vi "Kommunikation Geraetekennung.vi"(8 "error in (no error)":errorcluster caption="Fehler (Eingang, kein Fehler)", 11 "Steuerung PNS Eingang":refnum<class "Steuerung PNS.lvclass">) -> (0 "error out":errorcluster caption="Fehler (Ausgang)", 1 "Seriennummer":string, 2 "Gerätetype":string, 3 "Steuerung PNS Ausgang":refnum<class "Steuerung PNS.lvclass">)   [LabVIEW 2020, in "Steuerung PNS.lvclass"]
doc: "Kommuniziert mit der Steuerung, um die GeräteType auszulesen und in die Typenbezeichnung umzuwandeln, speichert diese im Objekt und stellt sie gelichzeitig als Output zur Verfügung.\nRIW"
uses:
  Steuerung PNS.lvclass
panel:
  out "SoftWare Vresion":string
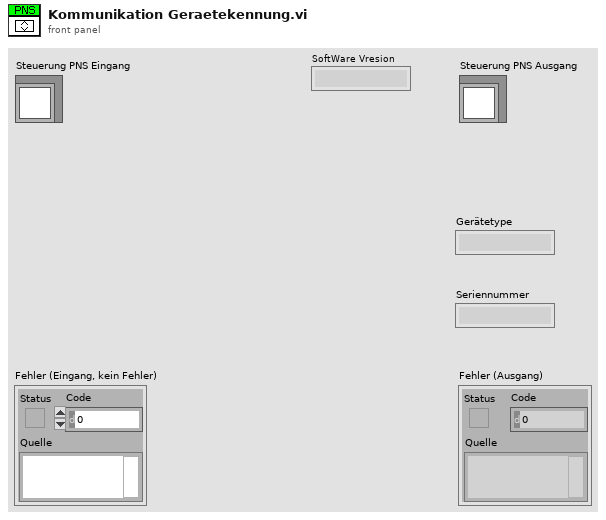
[diagram p1: front panel]
types:
  T1 = typedef "Steuerung PNS.lvclass/Adresse.ctl" = cluster{i32[][], i32}
  T2 = typedef "Steuerung PNS.lvclass/Werte.ctl" = cluster{"Adressen":u16[], "Werte":u16[]}
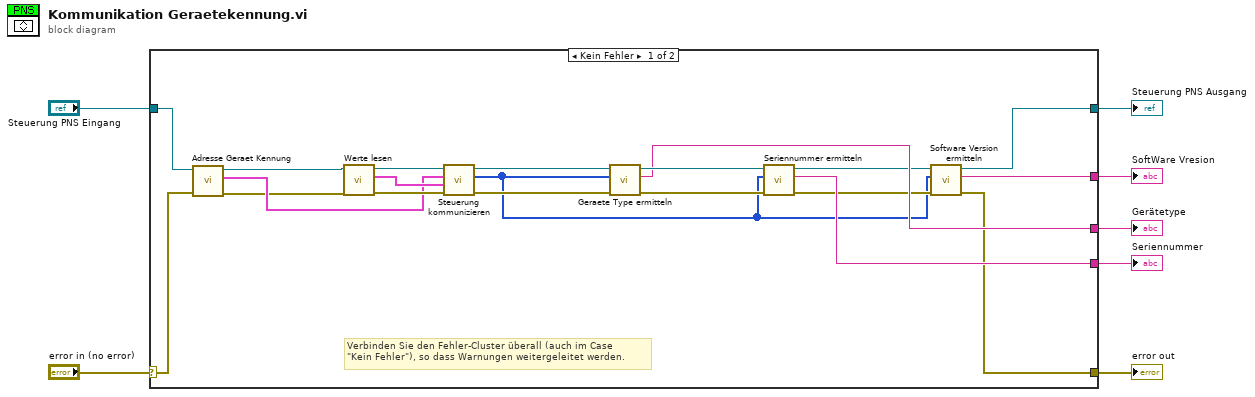
[diagram p0: block diagram]
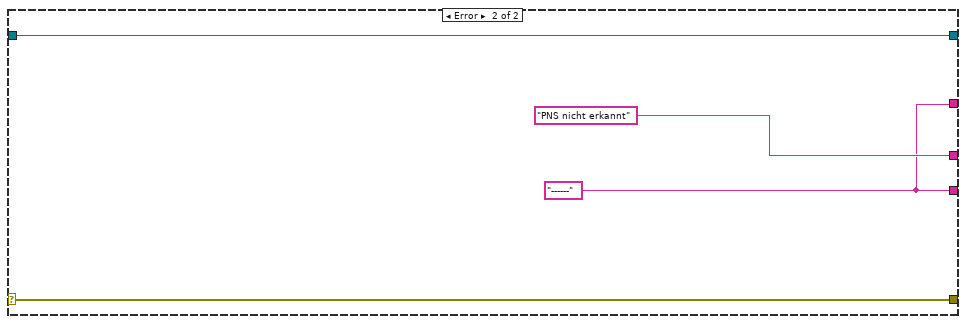
[diagram p2: hidden frame]
diagram:
  n1 = case shown="Kein Fehler" "error in (no error)" {
    selector: "error in (no error)" -> [w27 w31]
    tunnel: [w10 w31] -> w6
    tunnel: [w12 w30] -> w4
    tunnel: "Steuerung PNS Eingang" -> [w16 w30]
    tunnel: [w15 "PNS nicht erkannt" ("Gerätetype")] -> w3
    tunnel: [w14 w28] -> w2
    tunnel: [w8 w28] -> w1
    frame No Error {
      # "Verbinden Sie den Fehler-Cluster überall (auch im Case\n\"Kein Fehler\"), so dass Warnungen weitergeleitet werden."
      n2 = call-dynamic "Adresse Geraet Kennung.vi"("error in (no error)"=w27, "Steuerung PNS (Eingang)"=w16) -> ("error out"=w17:errorcluster, "Adressen"=w18:T1, "Steuerung PNS (Ausgang)"=w19:refnum<class "Steuerung PNS.lvclass">)  [unwired: 7 in]
      n3 = call-dynamic "Werte lesen.vi"("error in (no error)"=w17, "Steuerung PNS (Eingang)"=w19) -> ("error out"=w24:errorcluster, "Werte"=w22:T2, "Steuerung PNS (Ausgang)"=w26:refnum<class "Steuerung PNS.lvclass">)  [unwired: 7 in]
      n4 = call "Steuerung kommunizieren.vi"("Steuerung PNS Eingang"=w26, "Adressen"=w18, "Werte"=w22, "error in (no error)"=w24) -> ("Steuerung PNS Ausgang"=w25:refnum<class "Steuerung PNS.lvclass">, "Istwerte"=w9:u16[], "error out"=w23:errorcluster)  [unwired: 4 in]
      n5 = call "Geraete Type ermitteln.vi"("error in (no error)"=w23, "Istwerte"=w9, "Steuerung PNS Eingang"=w25) -> ("error out"=w20:errorcluster, "Gerätetype"=w15:string, "Steuerung PNS Ausgang"=w21:refnum<class "Steuerung PNS.lvclass">)  [unwired: 6 in]
      n6 = call "Seriennummer ermitteln.vi"("error in (no error)"=w20, "Istwerte"=w9, "Steuerung PNS Eingang"=w21) -> ("error out"=w11:errorcluster, "Seriennummer"=w14:string, "Steuerung PNS Ausgang"=w13:refnum<class "Steuerung PNS.lvclass">)  [unwired: 6 in]
      n7 = call "Software Version ermitteln.vi"("error in (no error)"=w11, "Istwerte"=w9, "Steuerung PNS Eingang"=w13) -> ("error out"=w10:errorcluster, "SoftWare Vresion"=w8:string, "Steuerung PNS Ausgang"=w12:refnum<class "Steuerung PNS.lvclass">)  [unwired: 6 in]
    }
    frame Error {
      w28 = "------"
    }
  }
  "error out" <- w6
  "Steuerung PNS Ausgang" <- w4
  "Gerätetype" <- w3
  "Seriennummer" <- w2
  "SoftWare Vresion" <- w1
